vi "Stage 1.2 myDAQ - Compartementlizing.vi"() -> ()   [LabVIEW 2018]
panel:
  out "error out":errorcluster
  out "Waveform Chart":waveform(dbl)(graph)
  in  "Stop":bool
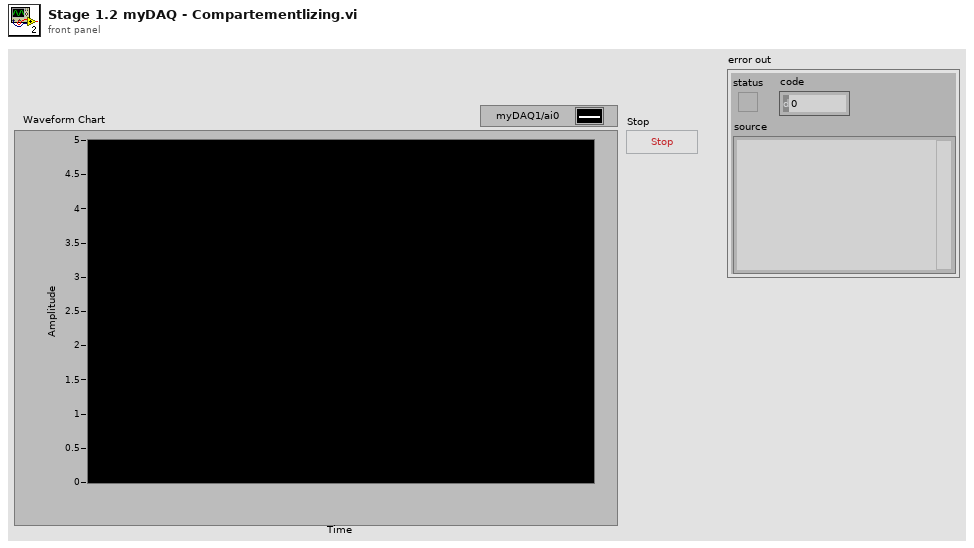
[diagram p1: front panel]
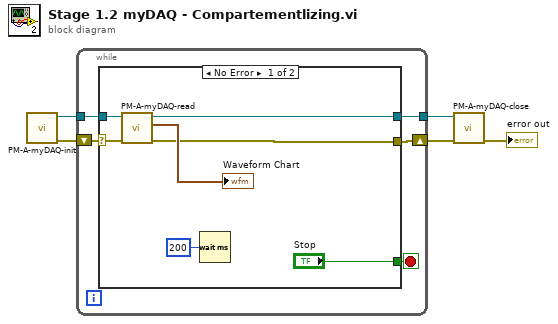
[diagram p0: block diagram]
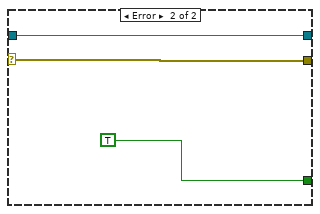
[diagram p2: hidden frame]
diagram:
  n1 = call "PM-A-myDAQ-init.vi"() -> ("error out"=w4:errorcluster, "Refnum out"=w3:refnum<k21>)  [unwired: 10 in]
  n2 = while {
    tunnel: w3 -> [w10]
    tunnel: [w8] -> w2
    shift-right: [w7] -> w1
    shift-left: w4 -> [w9]
    stop <- w6 stop-if-true
    n3 = case shown="No Error" w9 {
      selector: w9 -> [w16 w19]
      tunnel: w10 -> [w17 w18]
      tunnel: [w13 w18] -> w8
      tunnel: [w12 w19] -> w7
      tunnel: ["Stop" TRUE ("Stop")] -> w6
      frame No Error {
        n4 = call "PM-A-myDAQ-read.vi"("error in (no error)"=w16, "Refnum in"=w17) -> ("error out"=w12:errorcluster, "data"=→"Waveform Chart":waveform(dbl), "Refnum out"=w13:refnum<k21>)  [unwired: 7 in]
        n5 = Wait (ms)(milliseconds to wait=u32 200) -> ()  [unwired: 1 out]
      }
      frame Error {
      }
    }
  }
  n6 = call "PM-A-myDAQ-close.vi"("error in (no error)"=w1, "Refnum in"=w2) -> ("error out"=→"error out":errorcluster)  [unwired: 9 in]
